vi "RoboRIO_PanelSim_Global.vi"(0 "Menu":T3=enum."JSON update", 5 "Channel":i32, 7 "Value Set":bool, 9 "Numeric Value":dbl format="%#.4f", 11 "error in (no error)":errorcluster, 12 "String Value":string) -> (10 "roboRIO new":T1={"type"="roboRIO", "device"="", "name"="", "data"={">fpga_button"=FALSE, ">vin_voltage"=0.0, ">vin_current"=0.0, ">6v_voltage"=0.0, ">6v_current"=0.0, ">6v_active"=FALSE, ">6v_faults"=0.0, ">5v_voltage"=0.0, ">5v_current"=0.0, ">5v_active"=FALSE, ">5v_faults"=0.0, ">3v3_voltage"=0.0, ">3v3_current"=0.0, ">3v3_active"=FALSE, ">3v3_faults"=0.0}}, 15 "error out":errorcluster)   [LabVIEW 2019]
doc: "This is used to set and get the last motor output values. This is needed for simulation, since we cannot read these values from the hardware.\n\nThis software is licensed. Open the labview\\readme\\WPI Robotics Library Open Source License.txt file for more information."
uses:
  RoboRIO data proto.ctl
  RoboRIO proto.ctl
  RoboRIO Update Ops.ctl
panel:
  out "All Values":T1[](array[typedef])
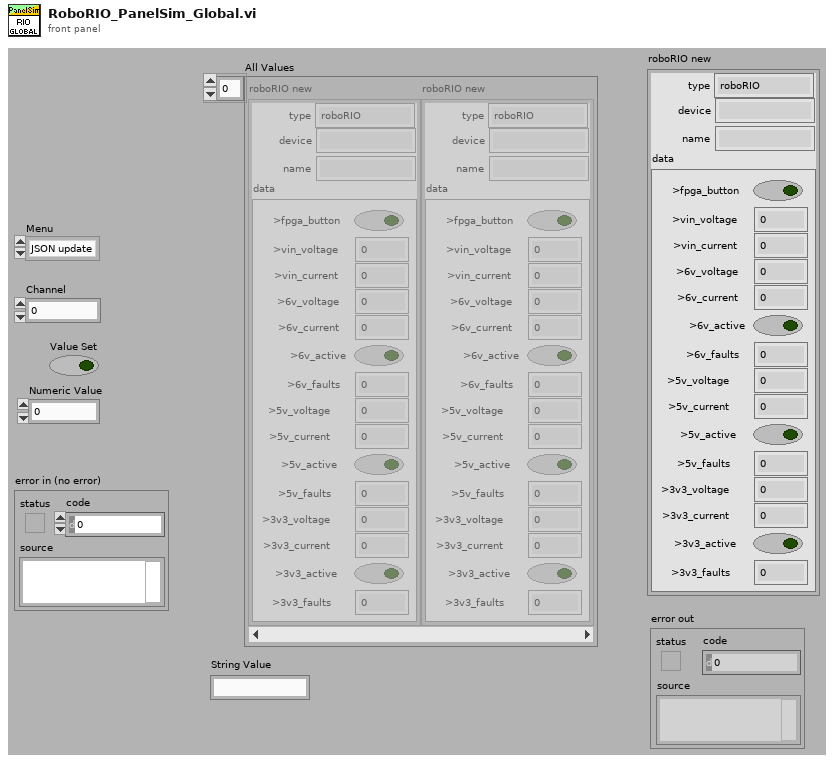
[diagram p1: front panel]
types:
  T1 = typedef "RoboRIO proto.ctl" = cluster{"type":string, "device":string, "name":string, "data":T2}
  T2 = typedef "RoboRIO data proto.ctl" = cluster{">fpga_button":bool, ">vin_voltage":dbl, ">vin_current":dbl, ">6v_voltage":dbl, ">6v_current":dbl, ">6v_active":bool, ">6v_faults":dbl, ">5v_voltage":dbl, ">5v_current":dbl, ">5v_active":bool, ">5v_faults":dbl, ">3v3_voltage":dbl, ">3v3_current":dbl, ">3v3_active":bool, ">3v3_faults":dbl}
  T3 = typedef "RoboRIO Update Ops.ctl" = enum16{"get", "JSON update", "set name", "transmit initial", "set fpga_button", "set vin_voltage", "set vin_current", "set 6v_voltage", "set 6v_current", "set 6v_active", "set 6v_faults", "set 5v_voltage", "set 5v_current", "set 5v_active", "set 5v_faults", "set 3v3_voltage", "set 3v3_current", "set 3v3_active", "set 3v3_faults", "reset"}
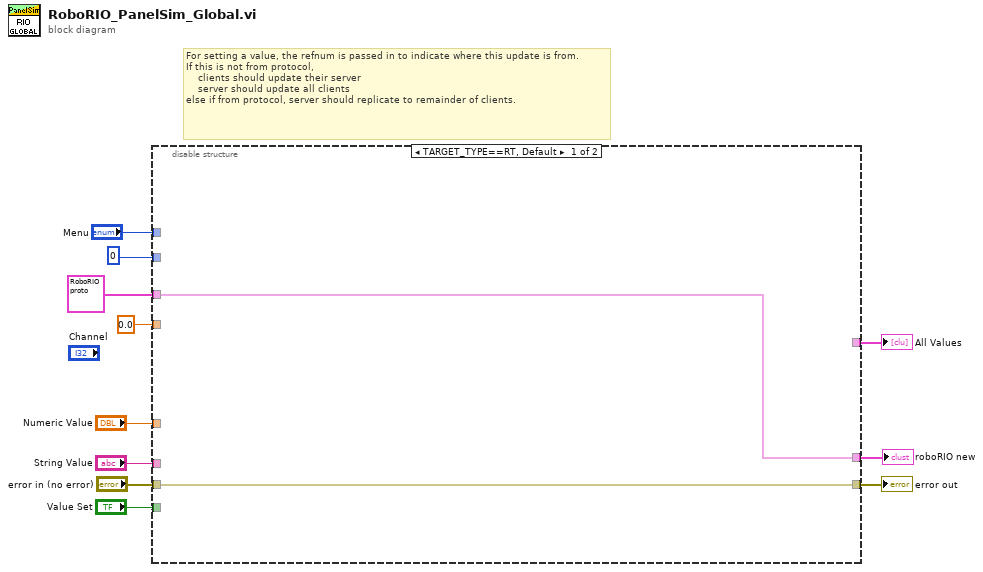
[diagram p0: block diagram]
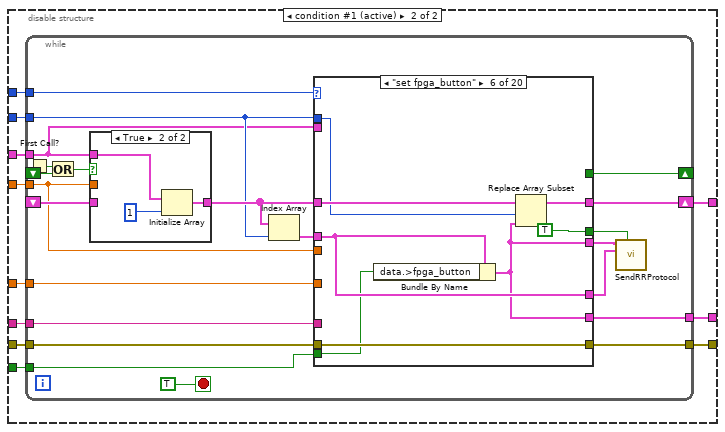
[diagram p2: hidden frame]
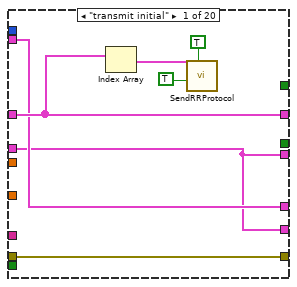
[diagram p3: hidden frame]
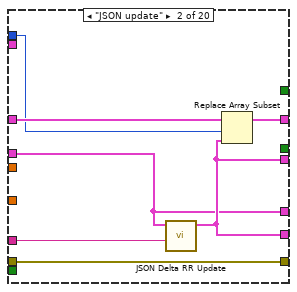
[diagram p4: hidden frame]
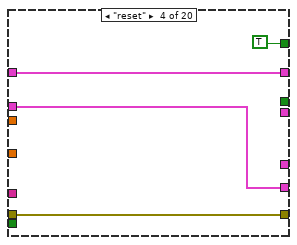
[diagram p6: hidden frame]
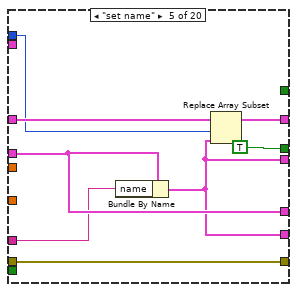
[diagram p7: hidden frame]
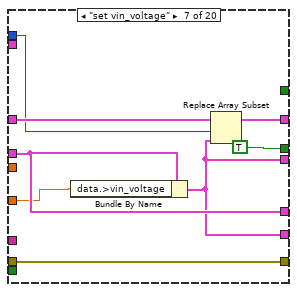
[diagram p8: hidden frame]
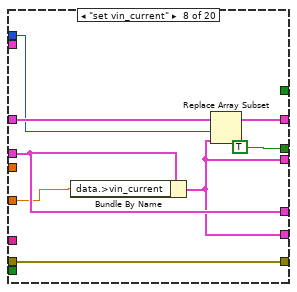
[diagram p9: hidden frame]
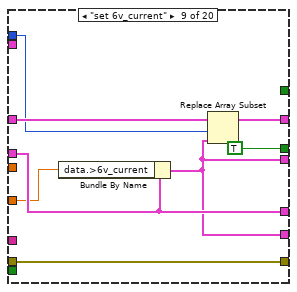
[diagram p10: hidden frame]
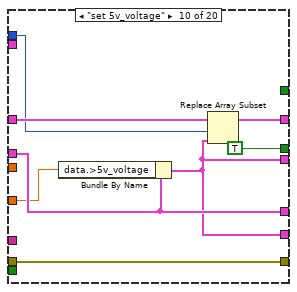
[diagram p11: hidden frame]
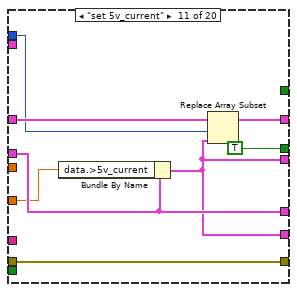
[diagram p12: hidden frame]
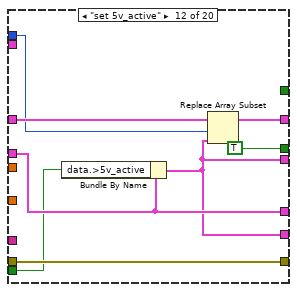
[diagram p13: hidden frame]
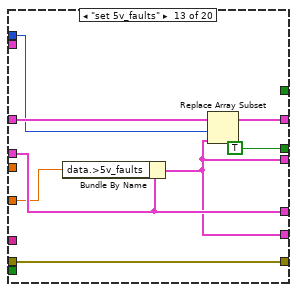
[diagram p14: hidden frame]
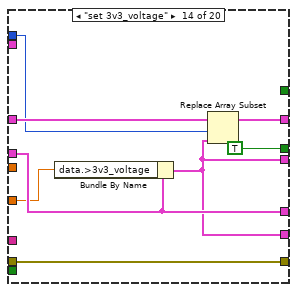
[diagram p15: hidden frame]
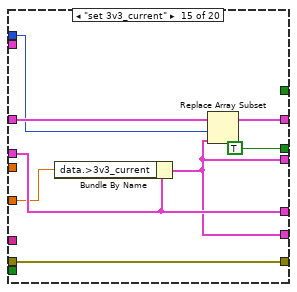
[diagram p16: hidden frame]
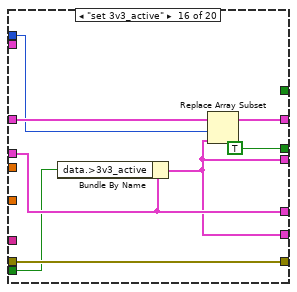
[diagram p17: hidden frame]
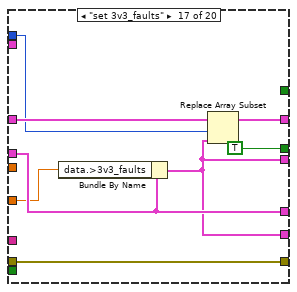
[diagram p18: hidden frame]
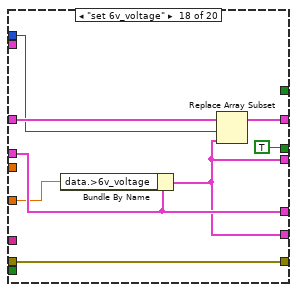
[diagram p19: hidden frame]
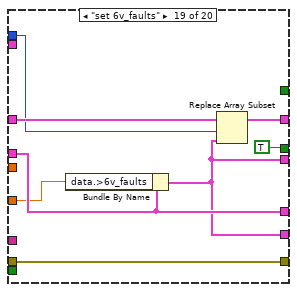
[diagram p20: hidden frame]
diagram:
  # "For setting a value, the refnum is passed in to indicate where this update is from.\nIf this is not from protocol,\n    clients should update their server\n    server should update all clients\nelse if from protocol, server should replicate to remainder of clients."
  n1 = disable-structure shown="TARGET_TYPE==RT, Default" {
    disable-tunnel: "Menu" -> [_ w24]
    disable-tunnel: [w13 w23] -> w10
    disable-tunnel: "error in (no error)" -> [w13 w22]
    disable-tunnel: [_ w21] -> w8
    disable-tunnel: 0.0 ("Output") -> [_ w20]
    disable-tunnel: 0 -> [_ w19]
    disable-tunnel: [w12 w18] -> w6
    disable-tunnel: T1 {"type"="RoboRIO", "device"="", "name"="", "data"={">fpga_button"=FALSE, ">vin_voltage"=0.0, ">vin_current"=0.0, ">6v_voltage"=0.0, ">6v_current"=0.0, ">6v_active"=FALSE, ">6v_faults"=0.0, ">5v_voltage"=0.0, ">5v_current"=0.0, ">5v_active"=FALSE, ">5v_faults"=0.0, ">3v3_voltage"=0.0, ">3v3_current"=0.0, ">3v3_active"=FALSE, ">3v3_faults"=0.0}} ("roboRIO new") -> [w12 w17]
    disable-tunnel: "String Value" -> [_ w16]
    disable-tunnel: "Numeric Value" -> [_ w15]
    disable-tunnel: "Value Set" -> [_ w14]
    frame condition #0 {
    }
    frame condition #1 (active) {
      n2 = while {
        tunnel: w22 -> [w43]
        shift-right: [w46] -> w21
        shift-left: _ -> [w39]
        tunnel: [w45] -> w18
        tunnel: w24 -> [w44]
        tunnel: [w42] -> w23
        tunnel: w19 -> [w37]
        tunnel: w20 -> [w38]
        tunnel: w17 -> [w36]
        tunnel: w16 -> [w35]
        tunnel: w15 -> [w34]
        tunnel: w14 -> [w33]
        shift-right: [w25] -> _
        shift-left: _ -> [w26]
        stop <- TRUE stop-if-true
        n3 = First Call?() -> (First Call?: T/F=w27:bool)
        n4 = Or(x=w27, y=w26) -> (x .or. y?=w28:bool)
        n5 = case shown="True" w28 {
          tunnel: [w196 w199] -> w40
          tunnel: w39 -> [w196 _]
          tunnel: w38 -> [_ _]
          tunnel: w36 -> [_ w198]
          frame False {
          }
          frame True {
            n6 = Initialize Array(w198, 1) -> (w199:T1[])
          }
        }
        n7 = Index Array(array=w40, index=w37) -> (element=w32:T1)
        n8 = case shown="\"set fpga_button\"" w44 {
          tunnel: [w52 w60 w63 w67 w75 w83 w91 w99 w107 w115 w123 w131 w139 w147 w155 w163 w171 w179 w187 w195] -> w46
          tunnel: w40 -> [w52 w58 w63 w67 w73 w81 w89 w97 w105 w113 w121 w129 w137 w145 w153 w161 w169 w177 w185 w193]
          tunnel: [w50 w56 w61 w65 w69 w77 w85 w93 w101 w109 w117 w125 w133 w141 w149 w157 w165 w173 w181 w189] -> w45
          tunnel: [w53 w59 w62 w66 w74 w82 w90 w98 w106 w114 w122 w130 w138 w146 w154 w162 w170 w178 w186 w194] -> w42
          tunnel: w43 -> [w53 w59 w62 w66 w74 w82 w90 w98 w106 w114 w122 w130 w138 w146 w154 w162 w170 w178 w186 w194]
          tunnel: w37 -> [_ w57 _ _ w71 w79 w87 w95 w103 w111 w119 w127 w135 w143 w151 w159 w167 w175 w183 w191]
          tunnel: w38 -> [_ _ _ _ _ _ _ _ _ _ _ _ _ _ _ _ _ _ _ _]
          tunnel: [w50 w56 _ _ w69 w77 w85 w93 w101 w109 w117 w125 w133 w141 w149 w157 w165 w173 w181 w189] -> w30
          tunnel: [w51 w54 _ _ w70 w78 w86 w94 w102 w110 w118 w126 w134 w142 w150 w158 w166 w174 w182 w190] -> w29
          tunnel: [_ _ _ _ TRUE TRUE TRUE TRUE TRUE TRUE TRUE TRUE TRUE TRUE TRUE TRUE TRUE TRUE TRUE TRUE] -> w31
          tunnel: w32 -> [w50 w54 w61 w65 w70 w78 w86 w94 w102 w110 w118 w126 w134 w142 w150 w158 w166 w174 w182 w190]
          tunnel: w36 -> [w51 _ _ _ _ _ _ _ _ _ _ _ _ _ _ _ _ _ _ _]
          tunnel: w35 -> [_ w55 _ _ w68 _ _ _ _ _ _ _ _ _ _ _ _ _ _ _]
          tunnel: w34 -> [_ _ _ _ _ _ w84 w92 w100 w108 w116 _ w132 w140 w148 _ w164 w172 w180 _]
          tunnel: w33 -> [_ _ _ _ _ w76 _ _ _ _ _ w124 _ _ _ w156 _ _ _ w188]
          tunnel: [_ _ _ TRUE _ _ _ _ _ _ _ _ _ _ _ _ _ _ _ _] -> w25
          frame "transmit initial" {
            n9 = Index Array(array=w52) -> (element=w47:T1)  [unwired: 1 in]
            n10 = call "SendRRProtocol.vi"("Send"=TRUE, "Initialize"=TRUE, "RR new"=w47) -> ()  [unwired: 9 in]
          }
          frame "JSON update" {
            n11 = call "JSON Delta RR Update.vi"("Delta JSON"=w55, "input"=w54) -> ("output"=w56:T1)  [unwired: 8 in, 1 out]
            n12 = Replace Array Subset(array=w58, new element=w56, index=w57) -> (w60:T1[])
          }
          frame "get" {
          }
          frame "reset" {
          }
          frame "set name" {
            n13 = Bundle By Name(cluster=w70, "name"=w68) -> (w69:T1)
            n14 = Replace Array Subset(array=w73, new element=w69, index=w71) -> (w75:T1[])
          }
          frame "set fpga_button" {
            n15 = Bundle By Name(cluster=w78, "data.>fpga_button"=w76) -> (w77:T1)
            n16 = Replace Array Subset(array=w81, new element=w77, index=w79) -> (w83:T1[])
          }
          frame "set vin_voltage" {
            n17 = Bundle By Name(cluster=w86, "data.>vin_voltage"=w84) -> (w85:T1)
            n18 = Replace Array Subset(array=w89, new element=w85, index=w87) -> (w91:T1[])
          }
          frame "set vin_current" {
            n19 = Bundle By Name(cluster=w94, "data.>vin_current"=w92) -> (w93:T1)
            n20 = Replace Array Subset(array=w97, new element=w93, index=w95) -> (w99:T1[])
          }
          frame "set 6v_current" {
            n21 = Bundle By Name(cluster=w102, "data.>6v_current"=w100) -> (w101:T1)
            n22 = Replace Array Subset(array=w105, new element=w101, index=w103) -> (w107:T1[])
          }
          frame "set 5v_voltage" {
            n23 = Bundle By Name(cluster=w110, "data.>5v_voltage"=w108) -> (w109:T1)
            n24 = Replace Array Subset(array=w113, new element=w109, index=w111) -> (w115:T1[])
          }
          frame "set 5v_current" {
            n25 = Bundle By Name(cluster=w118, "data.>5v_current"=w116) -> (w117:T1)
            n26 = Replace Array Subset(array=w121, new element=w117, index=w119) -> (w123:T1[])
          }
          frame "set 5v_active" {
            n27 = Bundle By Name(cluster=w126, "data.>5v_active"=w124) -> (w125:T1)
            n28 = Replace Array Subset(array=w129, new element=w125, index=w127) -> (w131:T1[])
          }
          frame "set 5v_faults" {
            n29 = Bundle By Name(cluster=w134, "data.>5v_faults"=w132) -> (w133:T1)
            n30 = Replace Array Subset(array=w137, new element=w133, index=w135) -> (w139:T1[])
          }
          frame "set 3v3_voltage" {
            n31 = Bundle By Name(cluster=w142, "data.>3v3_voltage"=w140) -> (w141:T1)
            n32 = Replace Array Subset(array=w145, new element=w141, index=w143) -> (w147:T1[])
          }
          frame "set 3v3_current" {
            n33 = Bundle By Name(cluster=w150, "data.>3v3_current"=w148) -> (w149:T1)
            n34 = Replace Array Subset(array=w153, new element=w149, index=w151) -> (w155:T1[])
          }
          frame "set 3v3_active" {
            n35 = Bundle By Name(cluster=w158, "data.>3v3_active"=w156) -> (w157:T1)
            n36 = Replace Array Subset(array=w161, new element=w157, index=w159) -> (w163:T1[])
          }
          frame "set 3v3_faults" {
            n37 = Bundle By Name(cluster=w166, "data.>3v3_faults"=w164) -> (w165:T1)
            n38 = Replace Array Subset(array=w169, new element=w165, index=w167) -> (w171:T1[])
          }
          frame "set 6v_voltage" {
            n39 = Bundle By Name(cluster=w174, "data.>6v_voltage"=w172) -> (w173:T1)
            n40 = Replace Array Subset(array=w177, new element=w173, index=w175) -> (w179:T1[])
          }
          frame "set 6v_faults" {
            n41 = Bundle By Name(cluster=w182, "data.>6v_faults"=w180) -> (w181:T1)
            n42 = Replace Array Subset(array=w185, new element=w181, index=w183) -> (w187:T1[])
          }
          frame "set 6v_active" {
            n43 = Bundle By Name(cluster=w190, "data.>6v_active"=w188) -> (w189:T1)
            n44 = Replace Array Subset(array=w193, new element=w189, index=w191) -> (w195:T1[])
          }
        }
        n45 = call "SendRRProtocol.vi"("Send"=w31, "RR old"=w29, "RR new"=w30) -> ()  [unwired: 9 in]
      }
    }
  }
  "error out" <- w10
  "All Values" <- w8
  "roboRIO new" <- w6
